vi "RobotStateMachine.vi"() -> ()   [LabVIEW 2018]
uses:
  Robot Global Data.vi
panel:
  in  "Claw Retract":bool
  in  "Claw Extend":bool
  in  "Claw Close":bool
  in  "Claw Open":bool
  in  "Shift":bool
  in  "Elevator Button Held":bool
  in  "stop":bool
  out "Robot State":T1(ring)
  out "Begin Hold":u32=172332208
  in  "Floor Intake":bool
  in  "Intake Cargo":bool
  in  "Intake Hatch":bool
  in  "Floor Cargo":bool
  in  "Stow":bool
  in  "Score Cargo":bool
  in  "Score Hatch":bool
  out "Wrist Angle":dbl
  out "Claw Extend Cmd":bool
  out "Kicker Out Cmd":bool
  out "Claw  Open Cmd":bool=TRUE
  in  "Wrist at Setpoint":bool
  in  "Game Piece Type":u16(ring) items=["Hatch", "Cargo"]
  out "Intake Out Cmd":bool
  in  "Elevator at Setpoint":bool
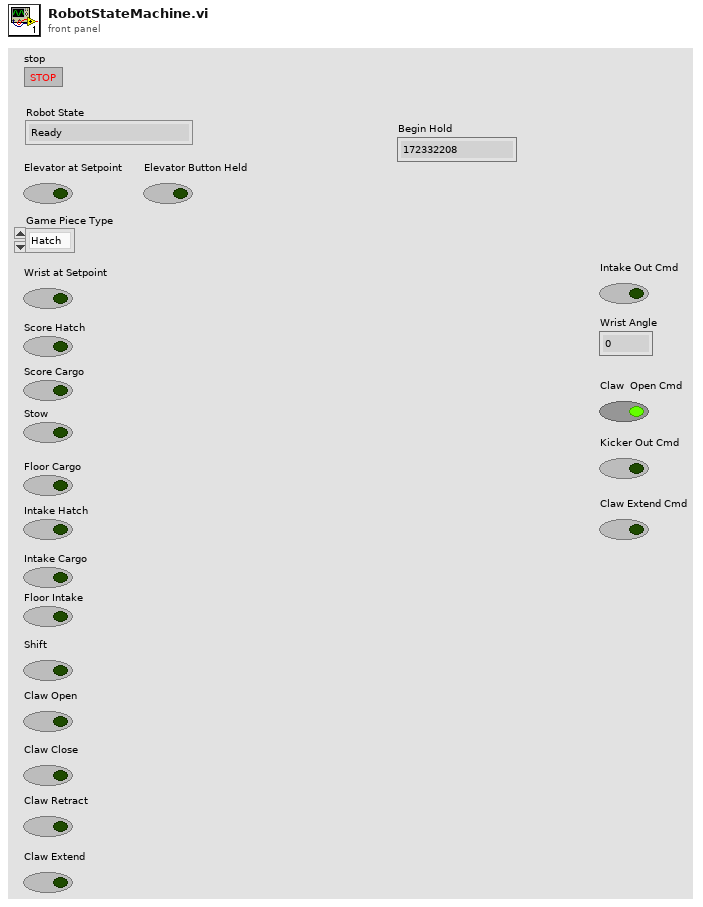
[diagram p1: front panel]
types:
  T1 = enum16{"Ready", "Stow", "Intake Hatch", "Intake Cargo", "Floor Cargo", "Go To Hatch", "Go To Cargo", "Score Hatch - Extend", "Score Hatch - Claw Closed", "Score Hatch - Retract", "Score Cargo - Extend", "Score Cargo - Claw Open", "Score Cargo - Retract"}
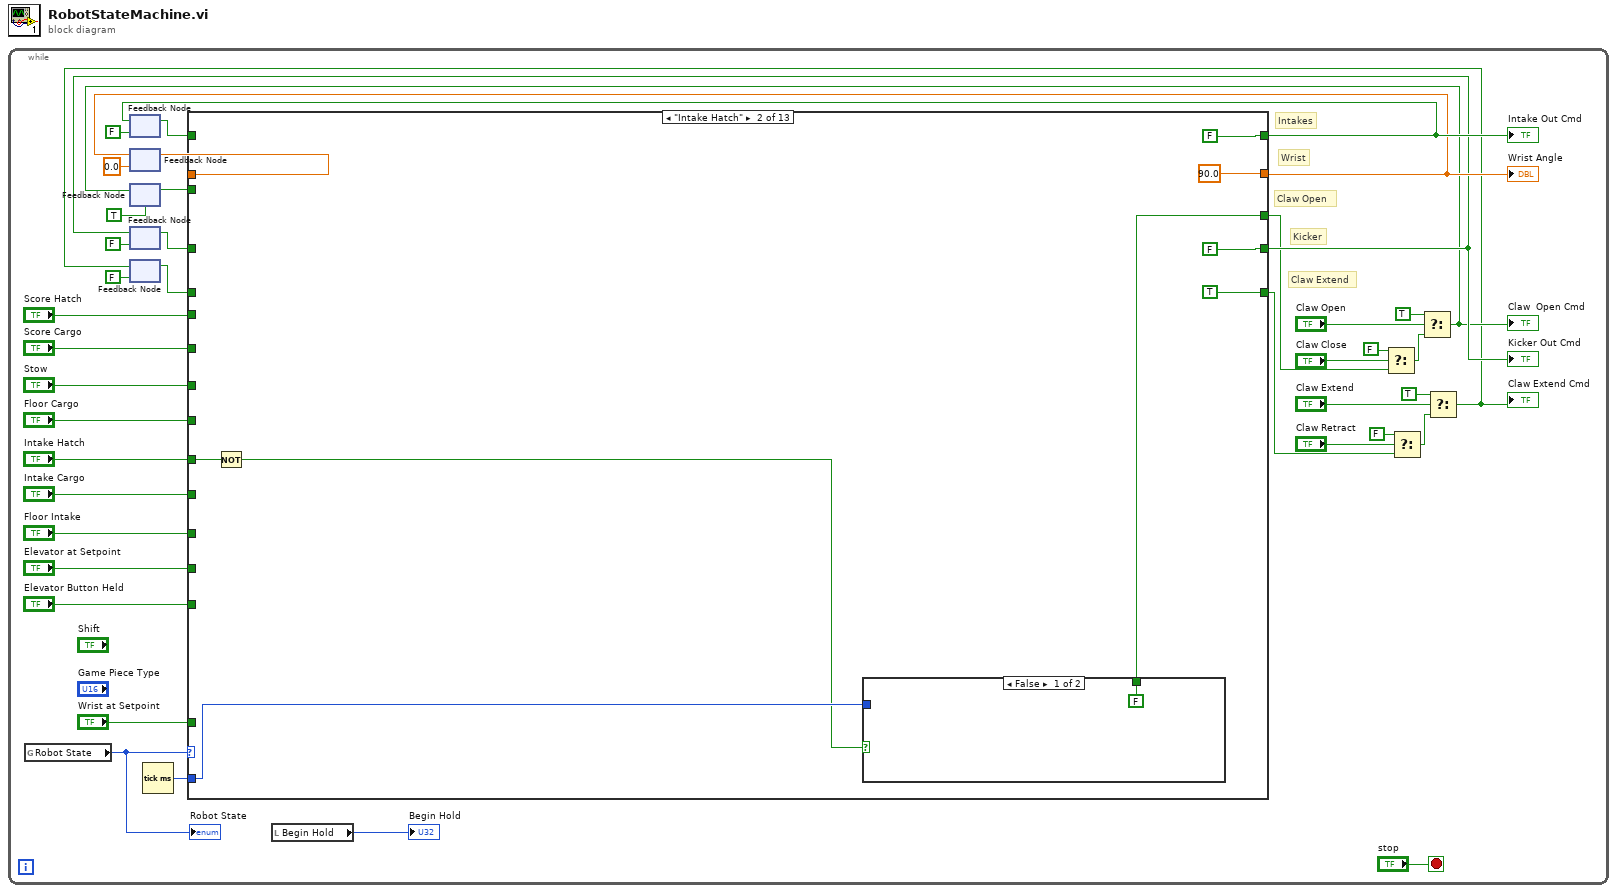
[diagram p0: block diagram]
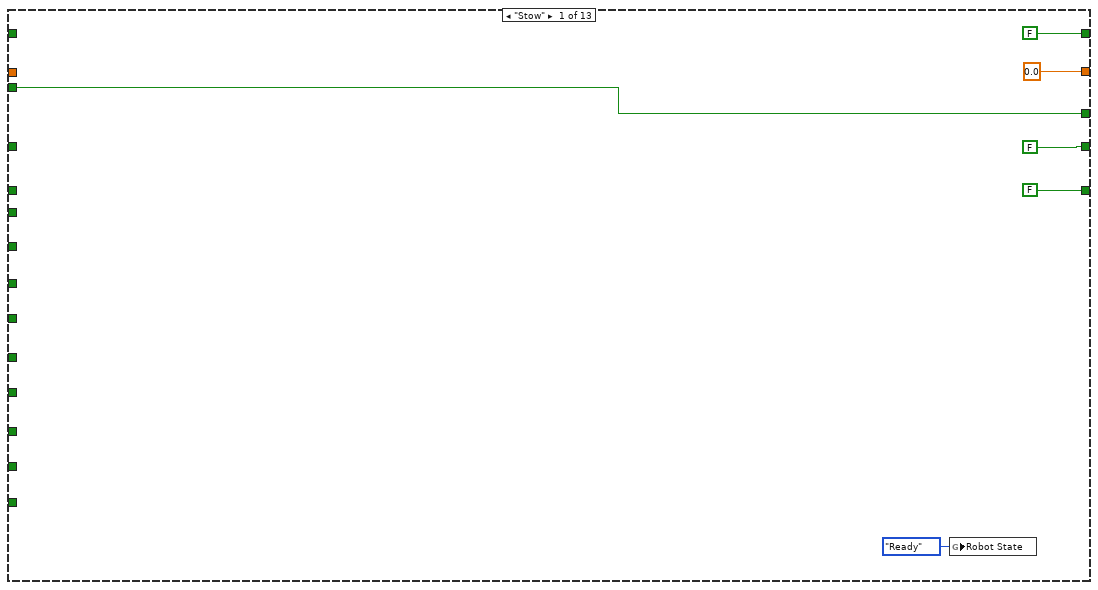
[diagram p2: hidden frame]
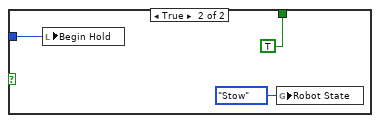
[diagram p3: hidden frame]
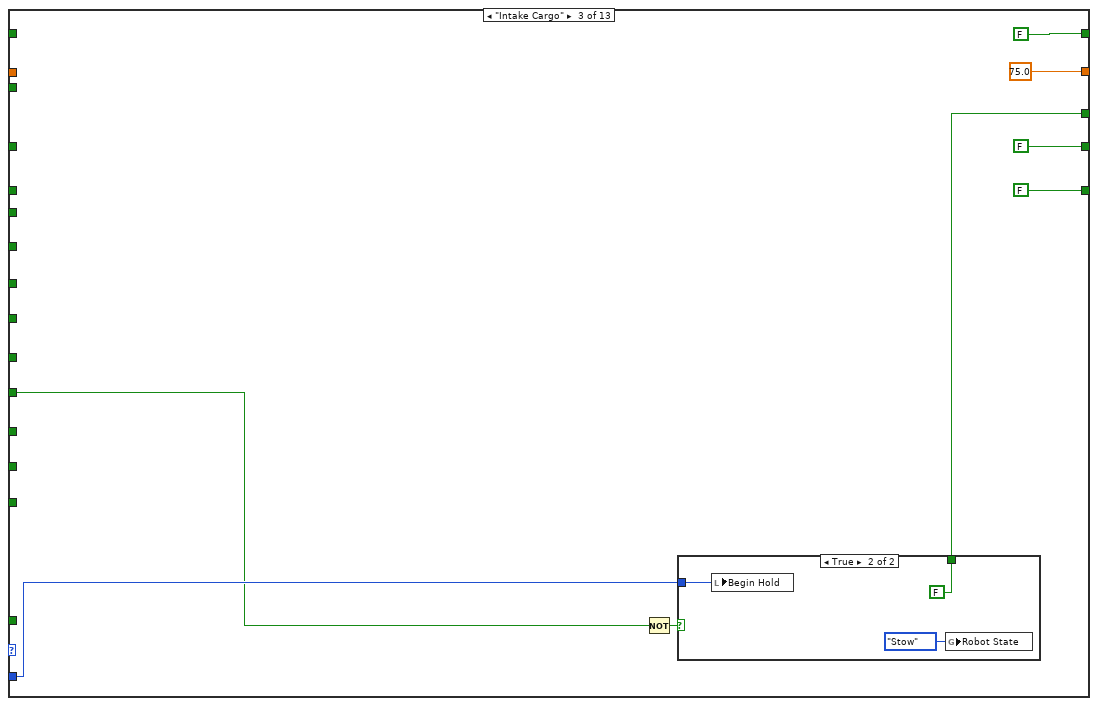
[diagram p4: hidden frame]
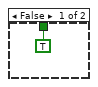
[diagram p5: hidden frame]
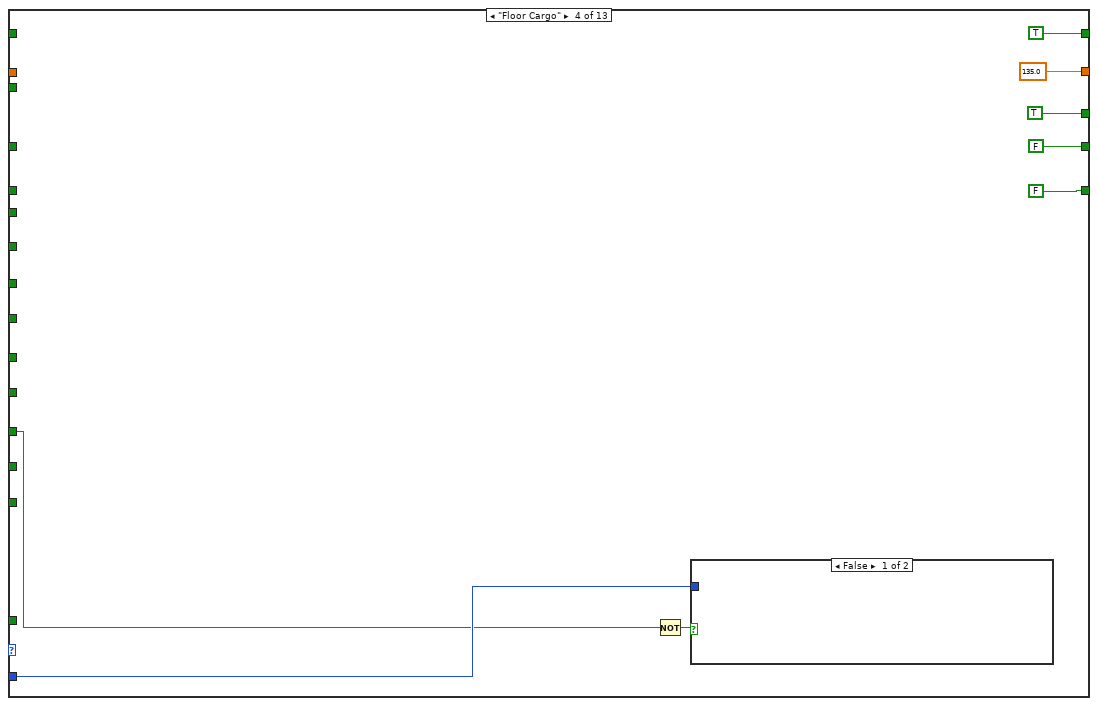
[diagram p6: hidden frame]
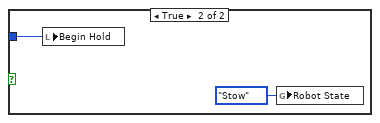
[diagram p7: hidden frame]
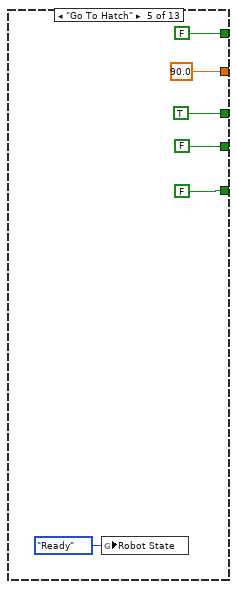
[diagram p8: hidden frame]
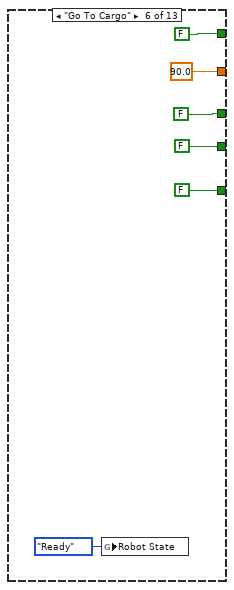
[diagram p9: hidden frame]
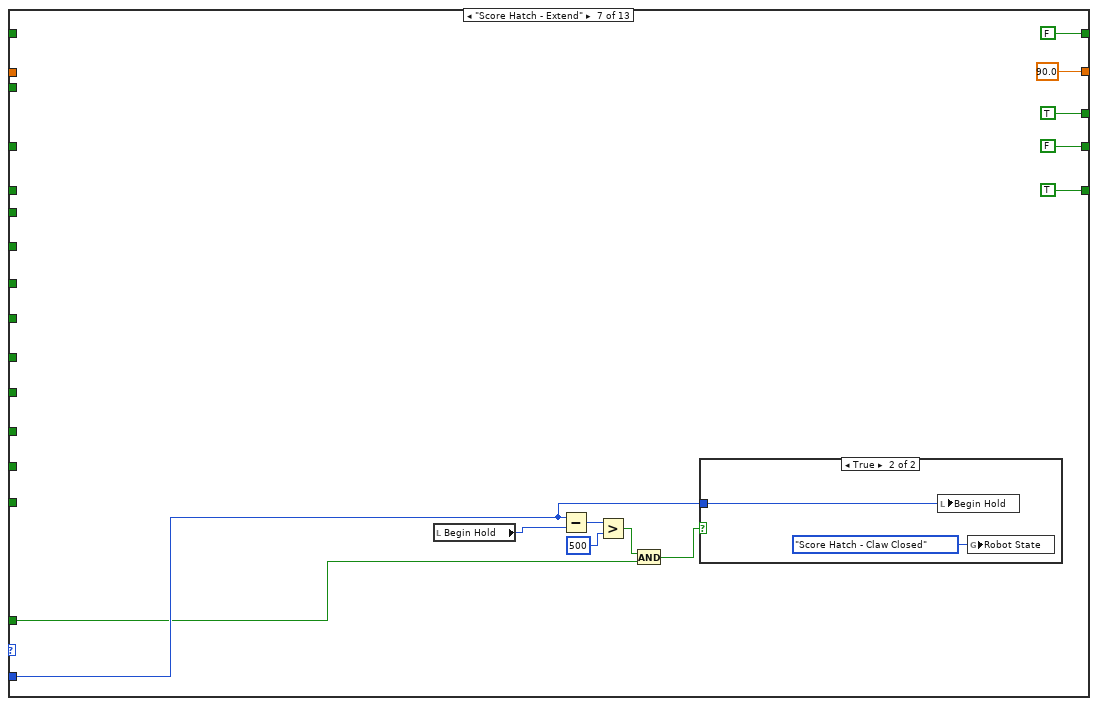
[diagram p10: hidden frame]
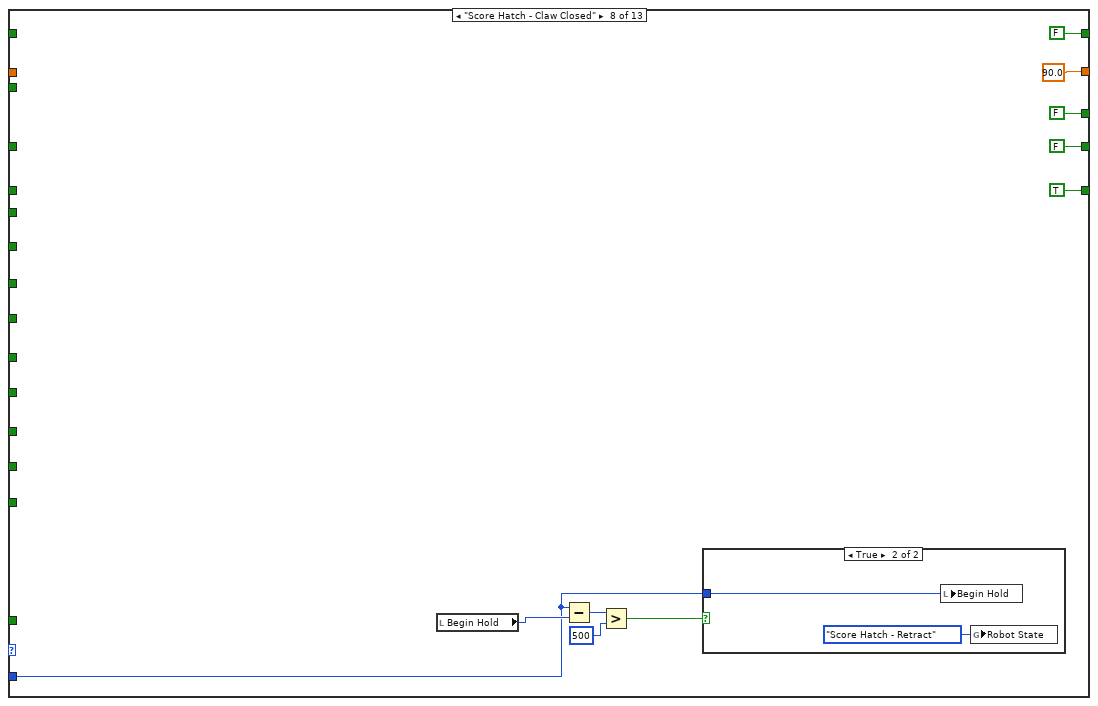
[diagram p12: hidden frame]
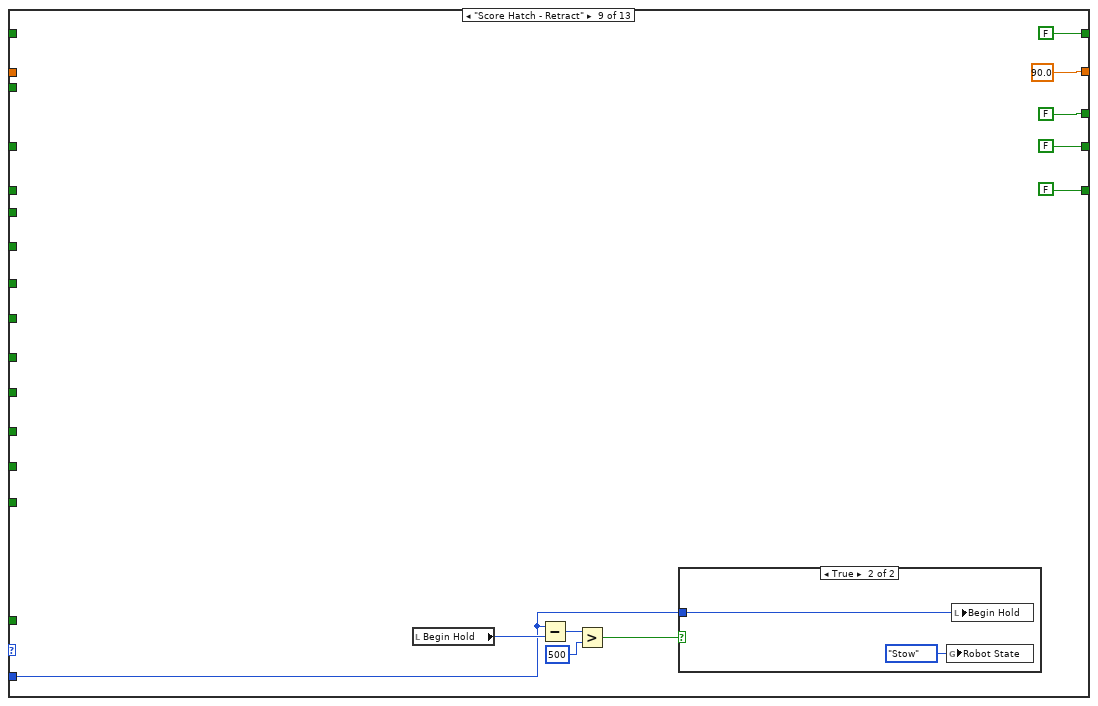
[diagram p14: hidden frame]
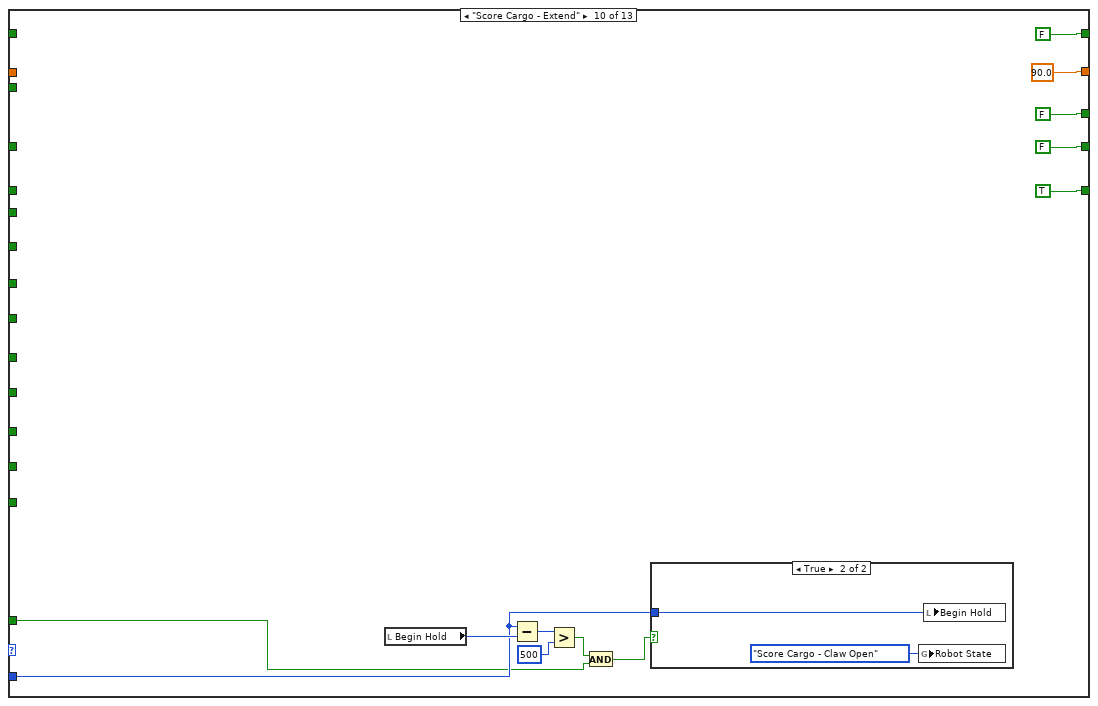
[diagram p16: hidden frame]
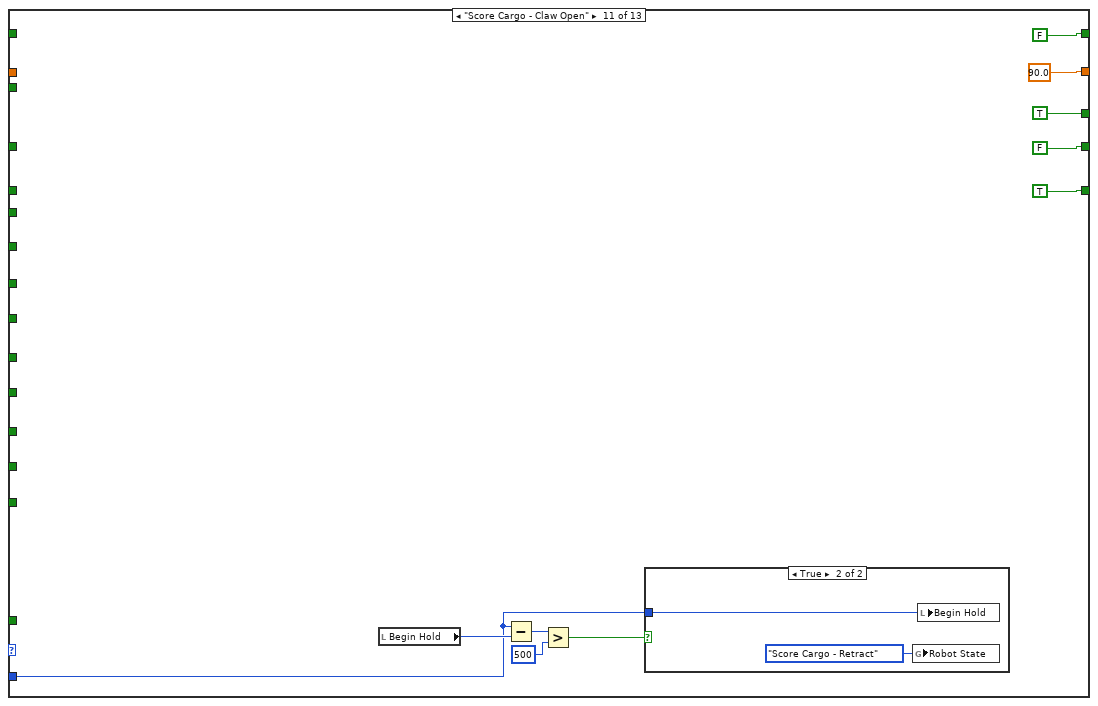
[diagram p18: hidden frame]
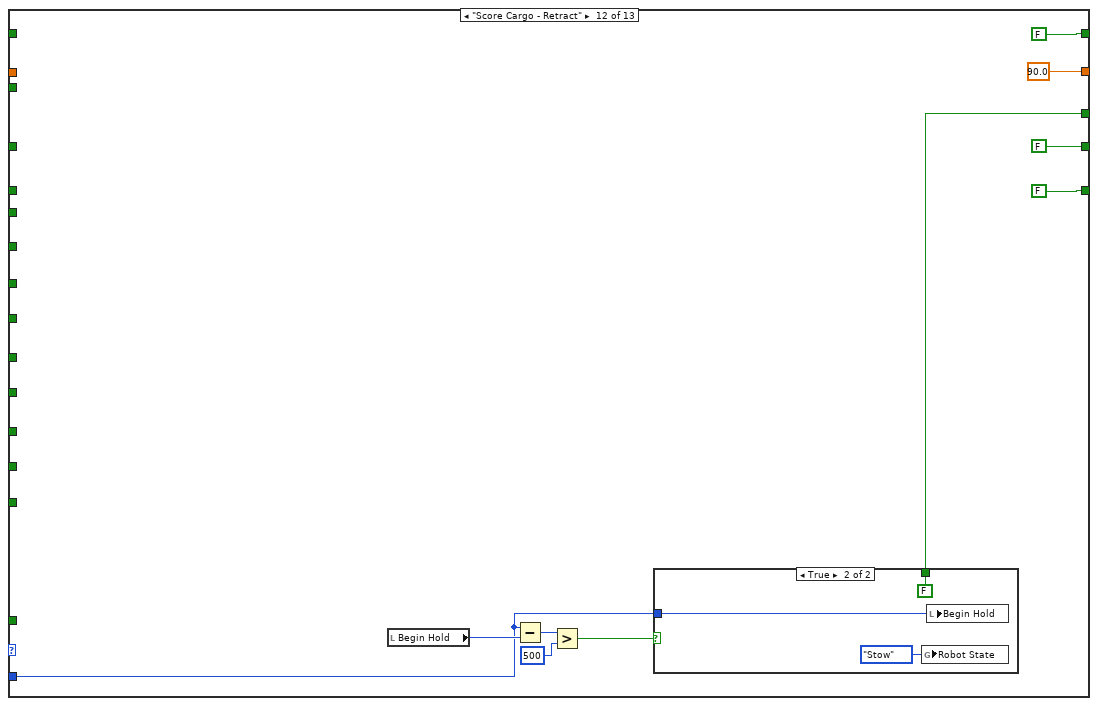
[diagram p20: hidden frame]
diagram:
  n1 = while {
    stop <- "stop" stop-if-true
    # "Claw Extend"
    # "Kicker"
    # "Claw Open"
    # "Wrist"
    # "Intakes"
    n2 = global read "Robot Global Data.vi" "Robot State"() -> (w41:T1)
    "Robot State" <- w41
    n3 = feedback #1(FALSE) -> (w35:bool)
    n4 = feedback #2(0.0) -> (w30:dbl)
    n5 = feedback #3(TRUE ("Claw  Open Cmd")) -> (w39:bool)
    n6 = feedback #4(FALSE) -> (w29:bool)
    n7 = feedback #5(FALSE) -> (w27:bool)
    n8 = Tick Count (ms)() -> (millisecond timer value=w26:u32)
    n9 = case shown="\"Intake Hatch\"" w41 {
      tunnel: [FALSE FALSE FALSE TRUE FALSE FALSE FALSE FALSE FALSE FALSE FALSE FALSE w189] -> w37
      tunnel: [FALSE FALSE FALSE FALSE FALSE FALSE FALSE FALSE FALSE FALSE FALSE FALSE w187] -> w32
      tunnel: [0.0 90.0 75.0 135.0 90.0 90.0 90.0 90.0 90.0 90.0 90.0 90.0 w188] -> w34
      tunnel: [FALSE TRUE FALSE FALSE FALSE FALSE TRUE TRUE FALSE TRUE TRUE FALSE w186] -> w8
      tunnel: [w44 w50 w60 TRUE ("Claw  Open Cmd") TRUE ("Claw  Open Cmd") FALSE ("Claw  Open Cmd") TRUE ("Claw  Open Cmd") FALSE ("Claw  Open Cmd") FALSE ("Claw  Open Cmd") FALSE ("Claw  Open Cmd") TRUE ("Claw  Open Cmd") w158 w190] -> w15
      tunnel: "Score Hatch" -> [_ _ _ _ _ _ _ _ _ _ _ _ w175]
      tunnel: "Score Cargo" -> [_ _ _ _ _ _ _ _ _ _ _ _ w176]
      tunnel: "Stow" -> [_ _ _ _ _ _ _ _ _ _ _ _ w199]
      tunnel: "Floor Cargo" -> [_ _ _ _ _ _ _ _ _ _ _ _ w177]
      tunnel: "Intake Hatch" -> [_ w49 _ _ _ _ _ _ _ _ _ _ w174]
      tunnel: "Intake Cargo" -> [_ _ w61 _ _ _ _ _ _ _ _ _ w173]
      tunnel: "Floor Intake" -> [_ _ _ w72 _ _ _ _ _ _ _ _ w172]
      tunnel: w39 -> [w44 _ _ _ _ _ _ _ _ _ _ _ w190]
      tunnel: w35 -> [_ _ _ _ _ _ _ _ _ _ _ _ w189]
      tunnel: w30 -> [_ _ _ _ _ _ _ _ _ _ _ _ w188]
      tunnel: w29 -> [_ _ _ _ _ _ _ _ _ _ _ _ w187]
      tunnel: w27 -> [_ _ _ _ _ _ _ _ _ _ _ _ w186]
      tunnel: w26 -> [_ w51 w63 w74 _ _ w97 w108 w120 w135 w146 w159 w184]
      tunnel: "Elevator Button Held" -> [_ _ _ _ _ _ _ _ _ _ _ _ w182]
      tunnel: "Elevator at Setpoint" -> [_ _ _ _ _ _ _ _ _ _ _ _ w181]
      tunnel: "Wrist at Setpoint" -> [_ _ _ _ _ _ w95 _ _ w132 _ _ _]
      frame "Stow" {
        n10 = global write "Robot Global Data.vi" "Robot State"(T1."Ready" ("Robot State")) -> ()
      }
      frame "Intake Hatch" {
        n11 = Not(x=w49) -> (.not. x?=w48:bool)
        n12 = case shown="False" w48 {
          tunnel: w51 -> [_ w58]
          tunnel: [FALSE TRUE] -> w50
          frame False {
          }
          frame True {
            n13 = local write "Begin Hold"(w58) -> ()
            n14 = global write "Robot Global Data.vi" "Robot State"(T1."Stow" ("Robot State")) -> ()
          }
        }
      }
      frame "Intake Cargo" {
        n15 = Not(x=w61) -> (.not. x?=w62:bool)
        n16 = case shown="True" w62 {
          tunnel: w63 -> [_ w70]
          tunnel: [TRUE FALSE] -> w60
          frame False {
          }
          frame True {
            n17 = local write "Begin Hold"(w70) -> ()
            n18 = global write "Robot Global Data.vi" "Robot State"(T1."Stow" ("Robot State")) -> ()
          }
        }
      }
      frame "Floor Cargo" {
        n19 = Not(x=w72) -> (.not. x?=w73:bool)
        n20 = case shown="False" w73 {
          tunnel: w74 -> [_ w80]
          frame False {
          }
          frame True {
            n21 = local write "Begin Hold"(w80) -> ()
            n22 = global write "Robot Global Data.vi" "Robot State"(T1."Stow" ("Robot State")) -> ()
          }
        }
      }
      frame "Go To Hatch" {
        n23 = global write "Robot Global Data.vi" "Robot State"(T1."Ready" ("Robot State")) -> ()
      }
      frame "Go To Cargo" {
        n24 = global write "Robot Global Data.vi" "Robot State"(T1."Ready" ("Robot State")) -> ()
      }
      frame "Score Hatch - Extend" {
        n25 = local read "Begin Hold"() -> (w100:u32)
        n26 = Subtract(x=w97, y=w100) -> (x-y=w99:u32)
        n27 = Greater?(x=w99, y=500) -> (0:w96:bool)
        n28 = And(x=w96, y=w95) -> (x .and. y?=w94:bool)
        n29 = case shown="True" w94 {
          tunnel: w97 -> [_ w106]
          frame False {
          }
          frame True {
            n30 = local write "Begin Hold"(w106) -> ()
            n31 = global write "Robot Global Data.vi" "Robot State"(T1."Score Hatch - Claw Closed" ("Robot State")) -> ()
          }
        }
      }
      frame "Score Hatch - Claw Closed" {
        n32 = local read "Begin Hold"() -> (w112:u32)
        n33 = Subtract(x=w108, y=w112) -> (x-y=w111:u32)
        n34 = Greater?(x=w111, y=500) -> (0:w109:bool)
        n35 = case shown="True" w109 {
          tunnel: w108 -> [_ w118]
          frame False {
          }
          frame True {
            n36 = local write "Begin Hold"(w118) -> ()
            n37 = global write "Robot Global Data.vi" "Robot State"(T1."Score Hatch - Retract" ("Robot State")) -> ()
          }
        }
      }
      frame "Score Hatch - Retract" {
        n38 = local read "Begin Hold"() -> (w124:u32)
        n39 = Subtract(x=w120, y=w124) -> (x-y=w123:u32)
        n40 = Greater?(x=w123, y=500) -> (0:w121:bool)
        n41 = case shown="True" w121 {
          tunnel: w120 -> [_ w130]
          frame False {
          }
          frame True {
            n42 = global write "Robot Global Data.vi" "Robot State"(T1."Stow" ("Robot State")) -> ()
            n43 = local write "Begin Hold"(w130) -> ()
          }
        }
      }
      frame "Score Cargo - Extend" {
        n44 = local read "Begin Hold"() -> (w138:u32)
        n45 = Subtract(x=w135, y=w138) -> (x-y=w137:u32)
        n46 = Greater?(x=w137, y=500) -> (0:w134:bool)
        n47 = And(x=w134, y=w132) -> (x .and. y?=w133:bool)
        n48 = case shown="True" w133 {
          tunnel: w135 -> [_ w144]
          frame False {
          }
          frame True {
            n49 = global write "Robot Global Data.vi" "Robot State"(T1."Score Cargo - Claw Open" ("Robot State")) -> ()
            n50 = local write "Begin Hold"(w144) -> ()
          }
        }
      }
      frame "Score Cargo - Claw Open" {
        n51 = local read "Begin Hold"() -> (w150:u32)
        n52 = Subtract(x=w146, y=w150) -> (x-y=w149:u32)
        n53 = Greater?(x=w149, y=500) -> (0:w147:bool)
        n54 = case shown="True" w147 {
          tunnel: w146 -> [_ w156]
          frame False {
          }
          frame True {
            n55 = global write "Robot Global Data.vi" "Robot State"(T1."Score Cargo - Retract" ("Robot State")) -> ()
            n56 = local write "Begin Hold"(w156) -> ()
          }
        }
      }
      frame "Score Cargo - Retract" {
        n57 = local read "Begin Hold"() -> (w163:u32)
        n58 = Subtract(x=w159, y=w163) -> (x-y=w162:u32)
        n59 = Greater?(x=w162, y=500) -> (0:w160:bool)
        n60 = case shown="True" w160 {
          tunnel: w159 -> [_ w170]
          tunnel: [TRUE ("Claw  Open Cmd") FALSE ("Claw  Open Cmd")] -> w158
          frame False {
          }
          frame True {
            n61 = global write "Robot Global Data.vi" "Robot State"(T1."Stow" ("Robot State")) -> ()
            n62 = local write "Begin Hold"(w170) -> ()
          }
        }
      }
      frame "Ready", Default {
        n63 = local write "Begin Hold"(w184) -> ()
        n64 = Not(x=w182) -> (.not. x?=w183:bool)
        n65 = And(x=w181, y=w183) -> (x .and. y?=w180:bool)
        n66 = And(x=w175, y=w180) -> (x .and. y?=w178:bool)
        n67 = And(x=w176, y=w180) -> (x .and. y?=w179:bool)
        n68 = Select(t=T1."Floor Cargo" ("Robot State"), s=w172, f=T1."Ready" ("Robot State")) -> (s? t:f=w192:T1)
        n69 = Select(t=T1."Intake Cargo" ("Robot State"), s=w173, f=w192) -> (s? t:f=w194:T1)
        n70 = Select(t=T1."Intake Hatch" ("Robot State"), s=w174, f=w194) -> (s? t:f=w197:T1)
        n71 = Select(t=T1."Floor Cargo" ("Robot State"), s=w177, f=w197) -> (s? t:f=w196:T1)
        n72 = Select(t=T1."Stow" ("Robot State"), s=w199, f=w196) -> (s? t:f=w202:T1)
        n73 = Select(t=T1."Score Cargo - Extend" ("Robot State"), s=w179, f=w202) -> (s? t:f=w204:T1)
        n74 = Select(t=T1."Score Hatch - Extend" ("Robot State"), s=w178, f=w204) -> (s? t:f=w191:T1)
        n75 = global write "Robot Global Data.vi" "Robot State"(w191) -> ()
      }
    }
    "Intake Out Cmd" <- w37
    "Kicker Out Cmd" <- w32
    "Wrist Angle" <- w34
    n76 = feedback-in #1(w37) -> ()
    n77 = feedback-in #2(w34) -> ()
    n78 = feedback-in #4(w32) -> ()
    n79 = local read "Begin Hold"() -> (→"Begin Hold":u32)
    n80 = Select(t=FALSE, s="Claw Close", f=w15) -> (s? t:f=w16:bool)
    n81 = Select(t=FALSE, s="Claw Retract", f=w8) -> (s? t:f=w13:bool)
    n82 = Select(t=TRUE, s="Claw Open", f=w16) -> (s? t:f=w14:bool)
    "Claw  Open Cmd" <- w14
    n83 = feedback-in #3(w14) -> ()
    n84 = Select(t=TRUE, s="Claw Extend", f=w13) -> (s? t:f=w7:bool)
    "Claw Extend Cmd" <- w7
    n85 = feedback-in #5(w7) -> ()
  }
